vi "Find Variable Indexes.vi"(8 "error in (no error)":errorcluster, 11 "all variables":refnum<k21>[](array[refnum])) -> (0 "error out":errorcluster, 2 "found?":bool, 3 "motor slave info":T1 {"nodeAddr" format="%.0x"})   [LabVIEW 2017, in "NI_Robotics_KUKA youBot Host.lvlib"]
uses:
  <vilib>/robotics/KUKA youBot/NI_Robotics_KUKA youBot Host.lvlib
  <vilib>/robotics/KUKA youBot/EtherCAT/Motor Slave Info.ctl
  <vilib>/robotics/KUKA youBot/EtherCAT/LowLevel/Mater Handler.ctl
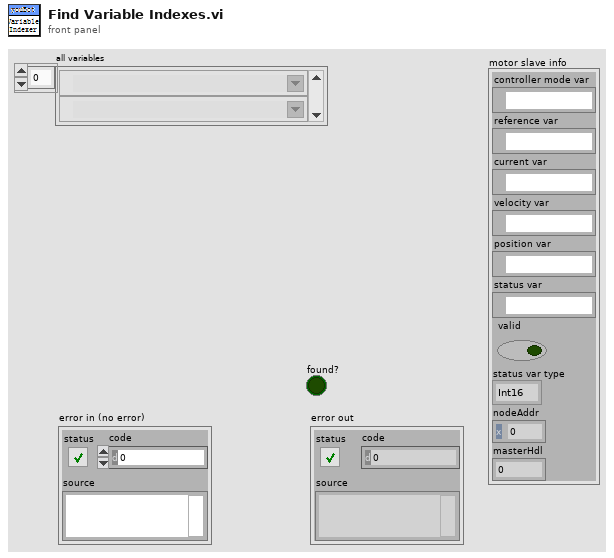
[diagram p1: front panel]
types:
  T1 = typedef "NI_Robotics_KUKA youBot Host.lvlib/Motor Slave Info.ctl" = cluster{"controller mode var":refnum<k21>, "reference var":refnum<k21>, "current var":refnum<k21>, "velocity var":refnum<k21>, "position var":refnum<k21>, "status var":refnum<k21>, "valid":bool, "status var type":enum16{"Int16", "Int32"}, "nodeAddr":u16, "masterHdl":T2}
  T2 = typedef "NI_Robotics_KUKA youBot Host.lvlib/Mater Handler.ctl" = i32
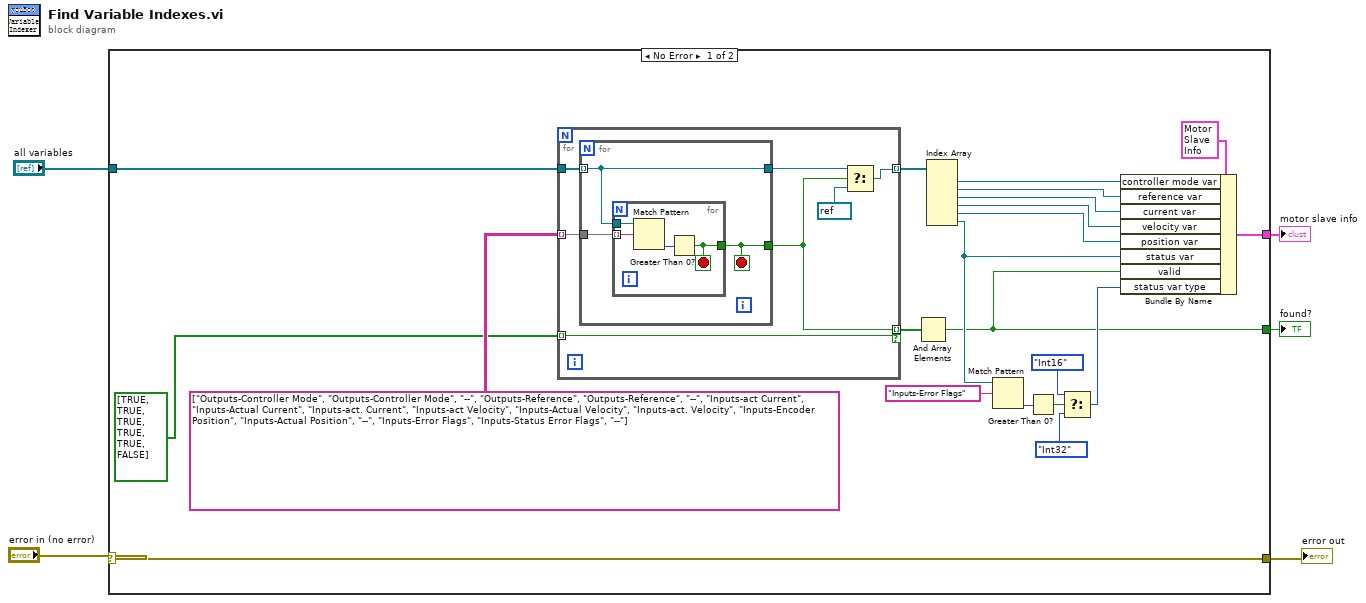
[diagram p0: block diagram]
diagram:
  n1 = case shown="No Error" "error in (no error)" {
    selector: "error in (no error)" -> [w25 w41]
    tunnel: [w26 _] -> w3
    tunnel: [w25 w41] -> w1
    tunnel: [w8 _] -> w2
    tunnel: "all variables" -> [w24 _]
    frame No Error {
      n2 = for {
        tunnel: w24 -> [w33]
        tunnel: [w28] -> w23 mode=indexing if=w27
        tunnel: [w31] -> w22 mode=indexing
        tunnel: string[][] [["Outputs-Controller Mode", "Outputs-Controller Mode", "--"], ["Outputs-Reference", "Outputs-Reference", "--"], ["Inputs-act Current", "Inputs-Actual Current", "Inputs-act. Current"], ["Inputs-act Velocity", "Inputs-Actual Velocity", "Inputs-act. Velocity"], ["Inputs-Encoder Position", "Inputs-Actual Position", "--"], ["Inputs-Error Flags", "Inputs-Status Error Flags", "--"]] -> [w29] mode=indexing
        tunnel: bool[] [TRUE, TRUE, TRUE, TRUE, TRUE, FALSE] -> [w27] mode=indexing
        n3 = for {
          tunnel: w33 -> [w35] mode=indexing
          tunnel: [w36] -> w28
          tunnel: [w35] -> w32
          tunnel: w29 -> [w34]
          stop <- w36 stop-if-true
          n4 = for {
            tunnel: w34 -> [w39] mode=indexing
            tunnel: [w38] -> w36
            tunnel: w35 -> [w37]
            stop <- w38 stop-if-true
            n5 = Match Pattern(string=w37, regular expression=w39) -> (offset past match=w40:i32)  [unwired: 1 in, 3 out]
            n6 = Greater Than 0?(x=w40) -> (x > 0?=w38:bool)
          }
        }
        n7 = Select(t=w32, s=w28, f=refnum<k21> refnum) -> (s? t:f=w31:refnum<k21>)
      }
      n8 = And Array Elements(Boolean array=w23) -> (logical AND=w8:bool)
      n9 = Index Array(array=w22) -> (element #1=w21:refnum<k21>, element #2=w20:refnum<k21>, element #3=w19:refnum<k21>, element #4=w18:refnum<k21>, element #5=w17:refnum<k21>, element #6=w14:refnum<k21>)  [unwired: 6 in]
      n10 = Match Pattern(string=w14, regular expression="Inputs-Error Flags") -> (offset past match=w15:i32)  [unwired: 1 in, 3 out]
      n11 = Greater Than 0?(x=w15) -> (x > 0?=w12:bool)
      n12 = Select(t=enum16{"Int16", "Int32"}."Int16" ("status var type"), s=w12, f=enum16{"Int16", "Int32"}."Int32" ("status var type")) -> (s? t:f=w9:enum16{"Int16", "Int32"})
      n13 = Bundle By Name(cluster=T1 {"controller mode var"="", "reference var"="", "current var"="", "velocity var"="", "position var"="", "status var"="", "valid"=FALSE, "status var type"=enum."Int16", "nodeAddr"=0, "masterHdl"=0} ("motor slave info"), "controller mode var"=w21, "reference var"=w20, "current var"=w19, "velocity var"=w18, "position var"=w17, "status var"=w14, "valid"=w8, "status var type"=w9) -> (w26:T1)
    }
    frame Error {
    }
  }
  "motor slave info" <- w3
  "found?" <- w2
  "error out" <- w1
